vi "TDK_Enable-Disable.vi"(7 "Enable PPS?":bool=TRUE, 8 "error":errorcluster, 11 "VISA":refnum<visa-resource-name>="COM1") -> (0 "error out":errorcluster)   [LabVIEW 2016]
panel:
  out "VISA out":refnum<visa-resource-name>
  in  "GEN Addr":i16=6
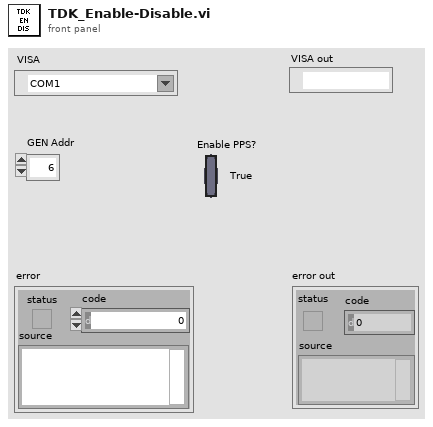
[diagram p1: front panel]
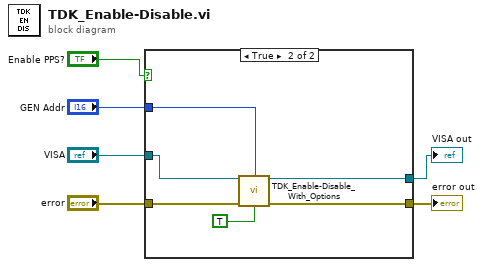
[diagram p0: block diagram]
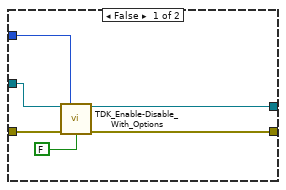
[diagram p2: hidden frame]
diagram:
  n1 = case shown="True" "Enable PPS?" {
    tunnel: "VISA" -> [w10 w17]
    tunnel: "error" -> [w9 w16]
    tunnel: [w12 w15] -> w3
    tunnel: [w11 w14] -> w2
    tunnel: "GEN Addr" -> [w7 w13]
    frame False {
      n2 = call "TDK_Enable-Disable_With_Options.vi"("VISA"=w10, "GEN Addr"=w7, "error"=w9, "Output On (T)"=FALSE) -> ("VISA out"=w12:refnum<visa-resource-name>, "error out"=w11:errorcluster)  [unwired: 10 in]
    }
    frame True {
      n3 = call "TDK_Enable-Disable_With_Options.vi"("VISA"=w17, "GEN Addr"=w13, "error"=w16, "Output On (T)"=TRUE) -> ("VISA out"=w15:refnum<visa-resource-name>, "error out"=w14:errorcluster)  [unwired: 10 in]
    }
  }
  "error out" <- w2
  "VISA out" <- w3
